vi "Files Copy to New Directory.vi"(6 "File Extensions to Error-Ignore (None)":string[](array[string]), 8 "error in (no error)":errorcluster, 9 "All Files":path[](array[path]), 10 "Base Folder":path, 11 "New Base Folder":path) -> (0 "error out":errorcluster, 2 "Copied?":bool)   [LabVIEW 2015]
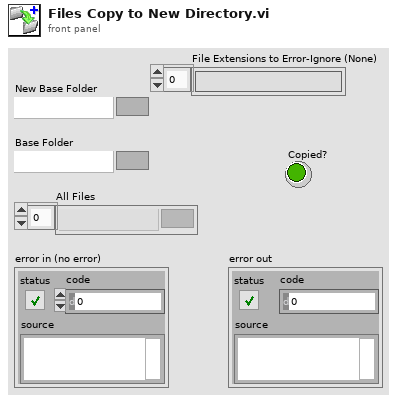
[diagram p1: front panel]
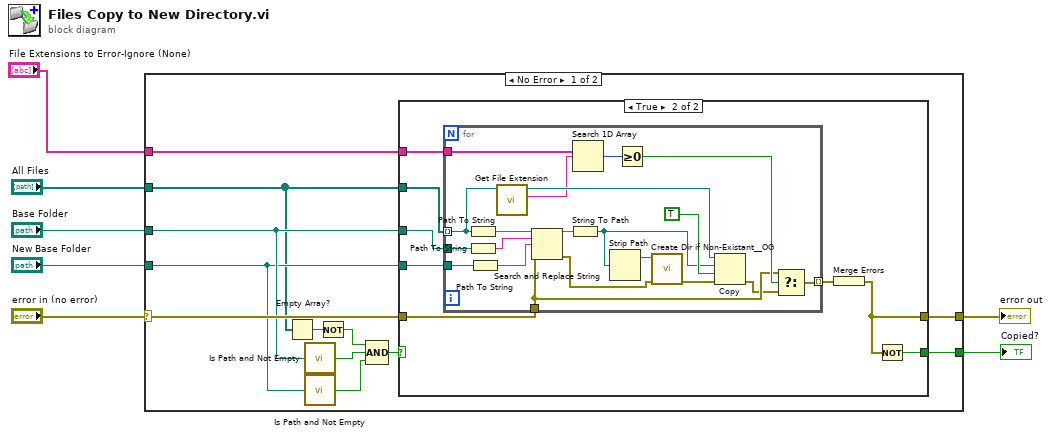
[diagram p0: block diagram]
diagram:
  n1 = case shown="No Error" "error in (no error)" {
    selector: "error in (no error)" -> [w19 w49]
    tunnel: [w18 w49] -> w6
    tunnel: "Base Folder" -> [w13 _]
    tunnel: "New Base Folder" -> [w12 _]
    tunnel: "All Files" -> [w10 _]
    tunnel: [w9 _] -> w2
    tunnel: "File Extensions to Error-Ignore (None)" -> [w8 _]
    frame No Error {
      n2 = Empty Array?(array=w10) -> (empty?=w11:bool)
      n3 = call <vilib>:"Is Path and Not Empty.vi"("path"=w13) -> ("Is Path and Not Empty?"=w14:bool)  [unwired: 4 in]
      n4 = call <vilib>:"Is Path and Not Empty.vi"("path"=w12) -> ("Is Path and Not Empty?"=w16:bool)  [unwired: 4 in]
      n5 = Not(x=w11) -> (.not. x?=w15:bool)
      n6 = Compound Arithmetic op=AND(w15, w14, w16) -> (w17:bool)
      n7 = case shown="True" w17 {
        tunnel: w13 -> [_ w28]
        tunnel: w10 -> [_ w27]
        tunnel: w19 -> [w20 w26]
        tunnel: [w20 w22] -> w18
        tunnel: w12 -> [_ w24]
        tunnel: [_ w23] -> w9
        tunnel: w8 -> [_ w21]
        frame False {
        }
        frame True {
          n8 = for {
            tunnel: w28 -> [w46]
            tunnel: w27 -> [w37] mode=indexing
            tunnel: [w29] -> w25 mode=indexing
            tunnel: w24 -> [w42]
            tunnel: w26 -> [w31]
            tunnel: w21 -> [w34]
            n9 = Path To String(path=w37) -> (string=w48:string)
            n10 = Path To String(path=w46) -> (string=w47:string)
            n11 = Path To String(path=w42) -> (string=w41:string)
            n12 = call <vilib>:"Get File Extension.vi"("file"=w37) -> ("lowercase file extension"=w35:string, "dup file"=w36:path)  [unwired: 6 in, 3 out]
            n13 = Search and Replace String(input string=w48, search string=w47, replace string=w41, error in=w31) -> (result string=w45:string, error out=w43:errorcluster)  [unwired: 4 in, 2 out]
            n14 = String To Path(string=w45) -> (path=w39:path)
            n15 = Search 1D Array(1D array=w34, element=w35) -> (index of element=w33:i32)  [unwired: 1 in]
            n16 = Strip Path(path=w39) -> (stripped path=w40:path)  [unwired: 1 out]
            n17 = Greater Or Equal To 0?(x=w33) -> (x >= 0?=w32:bool)
            n18 = call "Create Dir if Non-Existant__OG.vi"("error in (no error)"=w43, "Directory Path"=w40) -> ("error out"=w38:errorcluster)  [unwired: 7 in, 2 out]
            n19 = Copy(8:w38, 9:TRUE ("overwrite (F)"), 10:w39, 11:w36) -> (0:w30:errorcluster)  [unwired: 1 in, 2 out]
            n20 = Select(t=w31, s=w32, f=w30) -> (s? t:f=w29:errorcluster)
          }
          n21 = Merge Errors(w25) -> (w22:errorcluster)
          n22 = Not(x=w22) -> (.not. x?=w23:bool)
        }
      }
    }
    frame Error {
    }
  }
  "error out" <- w6
  "Copied?" <- w2
